vi "Teleop Pike Control.vi"(8 "Manipulator D-Pad":T1, 9 "Manipulator Buttons":T2, 10 "Driver D-Pad":T1, 11 "Driver Buttons":T2) -> ()   [LabVIEW 2014]
uses:
  Real-Life Controls/Button Cluster.ctl
  Real-Life Controls/D-Pad.ctl
  Pike Command.ctl
  Pike Mode.ctl
  Common Code/Change Detect Boolean.vi
  Robot Global Data.vi
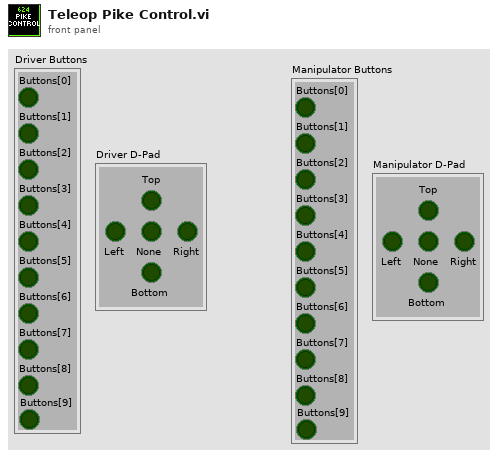
[diagram p1: front panel]
types:
  T1 = typedef "D-Pad.ctl" = cluster{"Top":bool, "Bottom":bool, "None":bool, "Right":bool, "Left":bool}
  T2 = typedef "Button Cluster.ctl" = cluster{"Buttons[0]":bool, "Buttons[1]":bool, "Buttons[2]":bool, "Buttons[3]":bool, "Buttons[4]":bool, "Buttons[5]":bool, "Buttons[6]":bool, "Buttons[7]":bool, "Buttons[8]":bool, "Buttons[9]":bool}
  T3 = typedef "Pike Mode.ctl" = enum16{"Idle", "Auto Down", "Auto Up", "Manual Down", "Manual Up"}
  T4 = typedef "Pike Command.ctl" = cluster{"Command":T3}
  T5 = typedef "Pike State.ctl" = enum16{"Up", "Down", "Going Up", "Going Down"}
  T6 = cluster{"Motor Out":dbl, "Current":dbl, "Limit Switch":bool, "Current Limit":bool, "State":T5, "Command":T3}
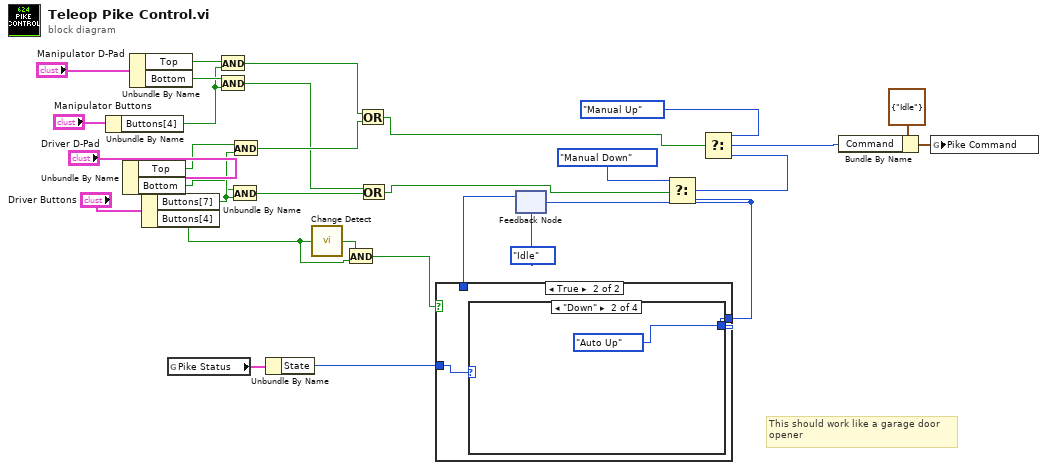
[diagram p0: block diagram]
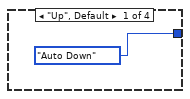
[diagram p3: hidden frame]
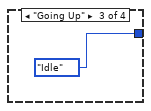
[diagram p4: hidden frame]
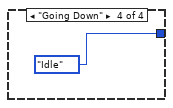
[diagram p5: hidden frame]
diagram:
  # "This should work like a garage door\nopener"
  n1 = Unbundle By Name("Manipulator Buttons") -> ("Buttons[4]"=w2:bool)
  n2 = Unbundle By Name("Driver D-Pad") -> ("Top"=w10:bool, "Bottom"=w9:bool)
  n3 = Unbundle By Name("Manipulator D-Pad") -> ("Top"=w6:bool, "Bottom"=w5:bool)
  n4 = Unbundle By Name("Driver Buttons") -> ("Buttons[7]"=w12:bool, "Buttons[4]"=w21:bool)
  n5 = global read "Robot Global Data.vi" "Pike Status"() -> (w16:T6)
  n6 = And(x=w6, y=w2) -> (x .and. y?=w3:bool)
  n7 = And(x=w5, y=w2) -> (x .and. y?=w7:bool)
  n8 = And(x=w9, y=w12) -> (x .and. y?=w11:bool)
  n9 = And(x=w10, y=w12) -> (x .and. y?=w13:bool)
  n10 = Unbundle By Name(w16) -> ("State"=w15:T5)
  n11 = call-poly "Change Detect.vi"("In"=w21) -> ("Changed?"=w22:bool)
  n12 = And(x=w22, y=w21) -> (x .and. y?=w17:bool)
  n13 = Or(x=w3, y=w13) -> (x .or. y?=w14:bool)
  n14 = Or(x=w7, y=w11) -> (x .or. y?=w8:bool)
  n15 = feedback #1(Pike_Mode."Idle" ("Command")) -> (w20:T3)
  n16 = case shown="True" w17 {
    tunnel: w20 -> [w31 _]
    tunnel: [w31 w33] -> w18
    tunnel: w15 -> [_ w32]
    frame False {
    }
    frame True {
      n17 = case shown="\"Down\"" w32 {
        tunnel: [Pike_Mode."Auto Down" ("Command") Pike_Mode."Auto Up" ("Command") Pike_Mode."Idle" ("Command") Pike_Mode."Idle" ("Command")] -> w33
        frame "Up", Default {
        }
        frame "Down" {
        }
        frame "Going Up" {
        }
        frame "Going Down" {
        }
      }
    }
  }
  n18 = feedback-in #1(w18) -> ()
  n19 = Select(t=Pike_Mode."Manual Down" ("Command"), s=w8, f=w18) -> (s? t:f=w25:T3)
  n20 = Select(t=Pike_Mode."Manual Up" ("Command"), s=w14, f=w25) -> (s? t:f=w23:T3)
  n21 = Bundle By Name(cluster=T4 {"Command"=enum."Idle"} ("Pike Command"), "Command"=w23) -> (w27:T4)
  n22 = global write "Robot Global Data.vi" "Pike Command"(w27) -> ()
